vi "EtherNet_IP Scan Registers.vi"(4 "error in":errorcluster, 5 "No of Elements":u8, 6 "Offset(N7:?)":u8, 7 "Connection Cluster":T1={"TCP Connection"=refnum, "Session"=[], "EtherNet/IP Device Address"="172.20.37.243"} {"Session" format="0x%02x"}) -> (0 "error out":errorcluster, 1 "Data Error":bool, 2 "Registers":u16[](array[numeric]), 3 "Connection Cluster Out":T1)   [LabVIEW 2020, in "EtherNet_IP_Lib.lvlib"]
uses:
  EtherNet_IP_Lib.lvlib
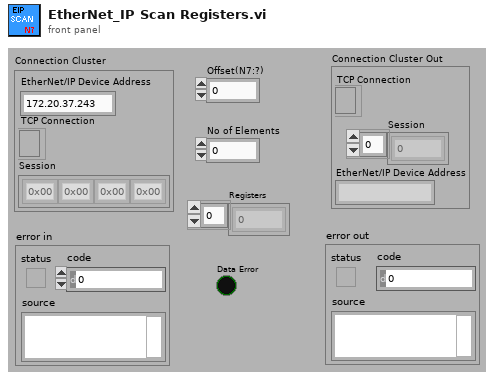
[diagram p1: front panel]
types:
  T1 = cluster{"TCP Connection":refnum<k5>, "Session":u8[], "EtherNet/IP Device Address":string}
  T2 = enum16{"Standard", "Buffered", "CRLF", "Immediate"}
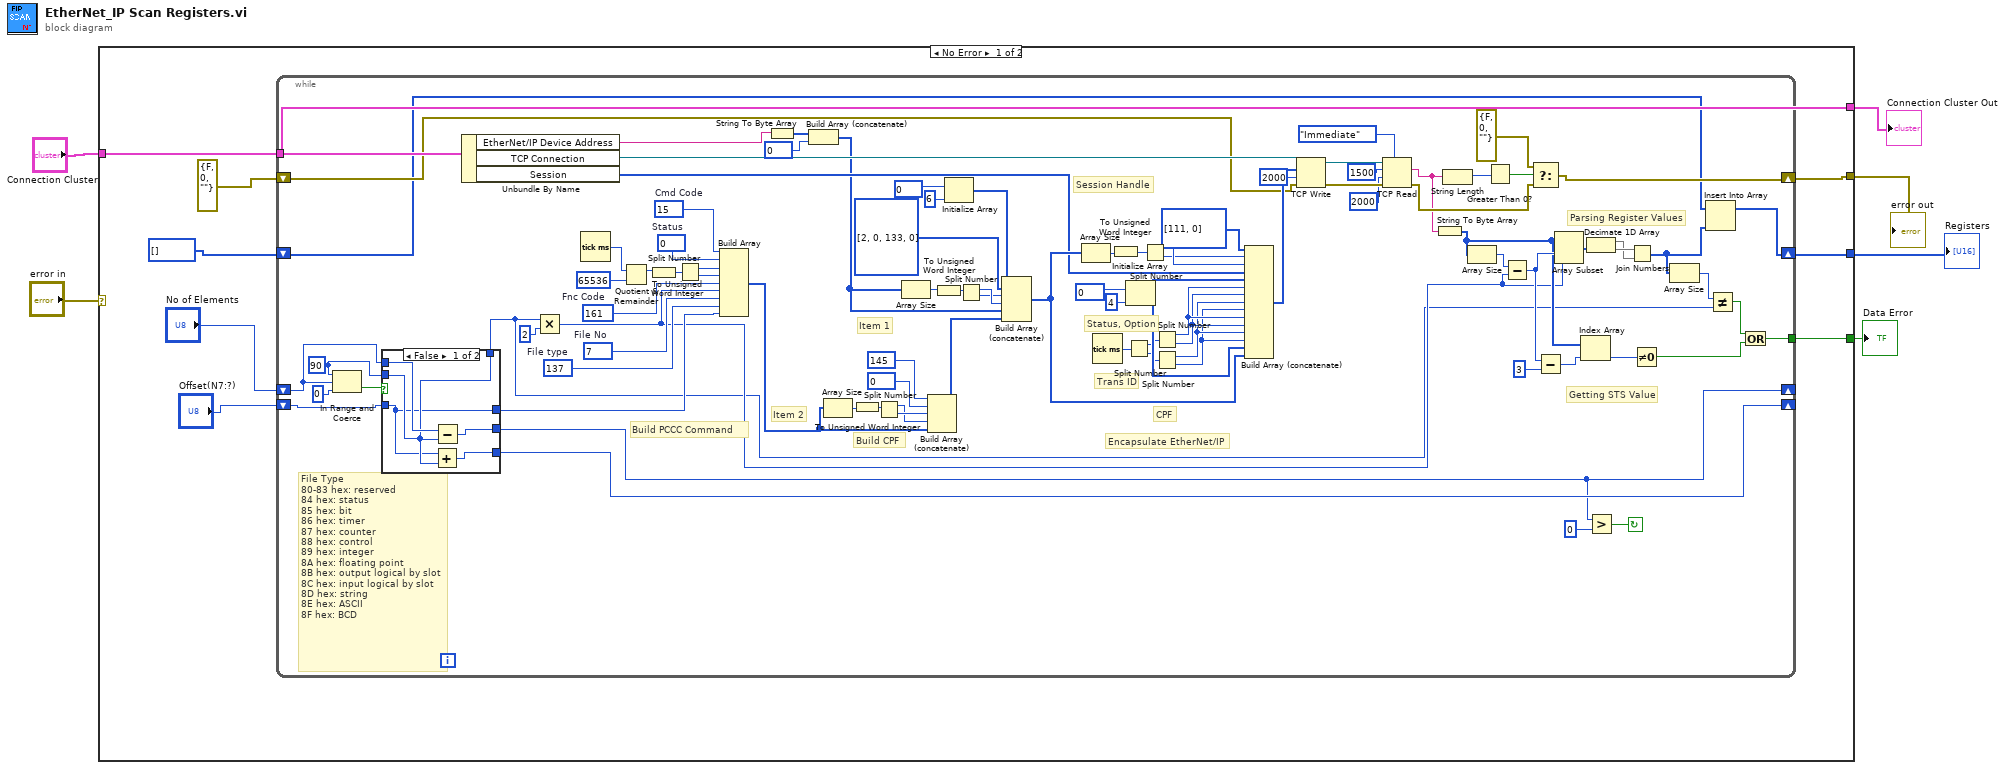
[diagram p0: block diagram]
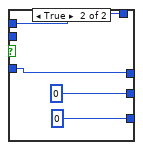
[diagram p2: hidden frame]
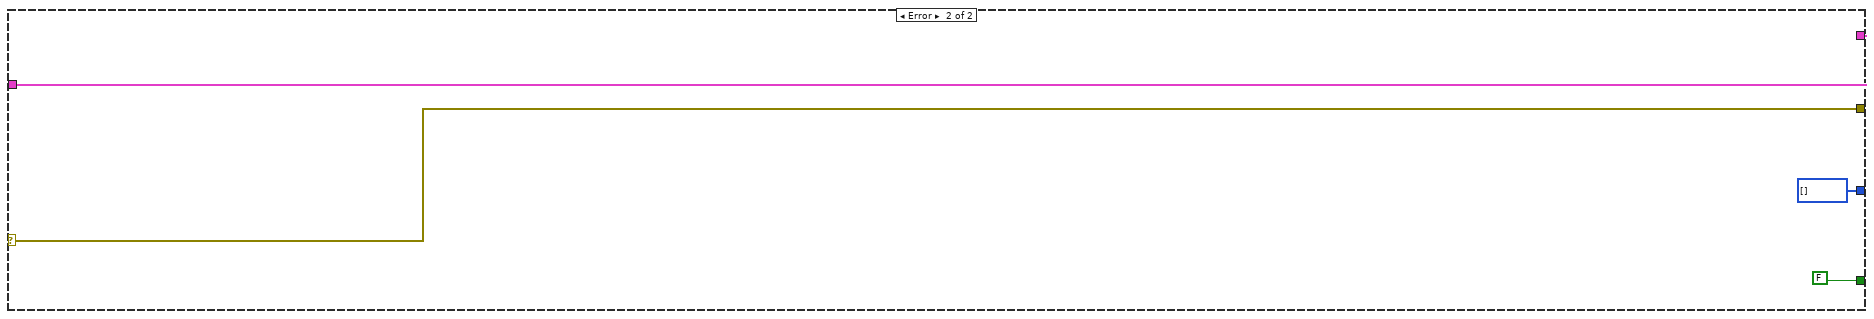
[diagram p3: hidden frame]
diagram:
  n1 = case shown="No Error" "error in" {
    selector: "error in" -> [_ w120]
    tunnel: "Connection Cluster" -> [w14 w119]
    tunnel: [w13 w120] -> w6
    tunnel: [w14 w119] -> w3
    tunnel: [w12 u16[] []] -> w2
    tunnel: [w11 FALSE] -> w1
    frame No Error {
      n2 = while {
        tunnel: w14 -> [w64]
        tunnel: [w32] -> w11
        shift-right: [w25] -> _
        shift-left: "No of Elements" -> [w28]
        shift-right: [w26] -> _
        shift-left: "Offset(N7:?)" -> [w27]
        shift-right: [w59] -> w13
        shift-left: errorcluster {"status"=FALSE, "code"=0, "source"=""} ("error out") -> [w21]
        shift-right: [w18] -> w12
        shift-left: u16[] [] -> [w19]
        stop <- w23 continue-if-true
        w22 = u8 90 ("upper limit")
        w50 = u8 137  # File type
        w51 = u8 7  # File No
        w52 = u8 161  # Fnc Code
        w100 = u8 0  # Status
        w99 = u8 15  # Cmd Code
        # "Getting STS Value"
        # "Parsing Register Values"
        # "File Type\n80-83 hex: reserved\n84 hex: status\n85 hex: bit\n86 hex: timer\n87 hex: counter\n88 hex: control\n89 hex: integer\n8A hex: floating point\n8B hex: output logical by slot\n8C hex: input logical by slot\n8D hex: string\n8E hex: ASCII\n8F hex: BCD"
        # "Build CPF"
        # "Trans ID"
        # "CPF"
        # "Status, Option"
        # "Session Handle"
        # "Item 2"
        # "Item 1"
        # "Encapsulate EtherNet/IP"
        # "Build PCCC Command"
        n3 = In Range and Coerce(upper limit=w22, x=w28, lower limit=u8 0) -> (In Range?=w29:bool)  [unwired: 1 out]
        n4 = case shown="False" w29 {
          tunnel: w28 -> [w112 w115]
          tunnel: w27 -> [w109 w116]
          tunnel: [w109 w116] -> w17
          tunnel: [w110 w115] -> w15
          tunnel: [w111 u8 0] -> w25
          tunnel: [w108 u8 0] -> w26
          tunnel: w22 -> [w110 _]
          frame False {
            n5 = Add(x=w109, y=w110) -> (x+y=w108:u8)
            n6 = Subtract(x=w112, y=w110) -> (x-y=w111:u8)
          }
          frame True {
          }
        }
        n7 = Unbundle By Name(w64) -> ("EtherNet/IP Device Address"=w65:string, "TCP Connection"=w104:refnum<k5>, "Session"=w75:u8[])
        n8 = Multiply(x=w15, y=u8 2) -> (x*y=w16:u8)
        n9 = Tick Count (ms)() -> (millisecond timer value=w95:u32)
        n10 = Quotient & Remainder(x=w95, y=u32 65536) -> (x-y*floor(x/y)=w97:u32)  [unwired: 1 out]
        n11 = To Unsigned Word Integer(number=w97) -> (unsigned 16bit integer=w98:u16)
        n12 = Split Number(x=w98) -> (hi(x)=w101:u8, lo(x)=w102:u8)
        n13 = Build Array(w99, w100, w101, w102, w52, w16, w51, w50, w17) -> (w54:u8[])
        n14 = String To Byte Array(string=w65) -> (unsigned byte array=w93:u8[])
        n15 = Build Array (concatenate)(w93, u8 0 ("Status")) -> (w57:u8[])
        n16 = Array Size(array=w54) -> (size(s)=w92:i32)
        n17 = To Unsigned Word Integer(number=w92) -> (unsigned 16bit integer=w91:u16)
        n18 = Split Number(x=w91) -> (hi(x)=w89:u8, lo(x)=w90:u8)
        n19 = Array Size(array=w57) -> (size(s)=w55:i32)
        n20 = Build Array (concatenate)(u8 145 ("Status"), u8 0 ("Status"), w90, w89, w54) -> (w53:u8[])
        n21 = To Unsigned Word Integer(number=w55) -> (unsigned 16bit integer=w56:u16)
        n22 = Initialize Array(u8 0 ("Status"), 6 ("dimension size")) -> (w84:u8[])
        n23 = Split Number(x=w56) -> (hi(x)=w47:u8, lo(x)=w46:u8)
        n24 = Build Array (concatenate)(w84, u8[] [2, 0, 133, 0], w46, w47, w57, w53) -> (w76:u8[])
        n25 = Array Size(array=w76) -> (size(s)=w82:i32)
        n26 = Tick Count (ms)() -> (millisecond timer value=w74:u32)
        n27 = To Unsigned Word Integer(number=w82) -> (unsigned 16bit integer=w83:u16)
        n28 = Split Number(x=w74) -> (hi(x)=w73:u16, lo(x)=w72:u16)
        n29 = Initialize Array(u8 0 ("Status"), 4 ("dimension size")) -> (w77:u8[])
        n30 = Split Number(x=w83) -> (hi(x)=w81:u8, lo(x)=w80:u8)
        n31 = Split Number(x=w73) -> (hi(x)=w71:u8, lo(x)=w70:u8)
        n32 = Split Number(x=w72) -> (hi(x)=w69:u8, lo(x)=w68:u8)
        n33 = Build Array (concatenate)(u8[] [111, 0], w80, w81, w75, w77, w71, w70, w69, w68, w71, w70, w69, w68, w77, w76) -> (w67:u8[])
        n34 = TCP Write(connection ID=w104, data in=w67, error in (no error)=w21, 9:2000 ("timeout ms (25000)")) -> (connection ID out=w106:refnum<k5>, error out=w107:errorcluster)  [unwired: 1 out]
        n35 = TCP Read(connection ID=w106, bytes to read=1500, error in (no error)=w107, 7:T2."Immediate" ("mode (standard)"), 9:2000 ("timeout ms (25000)")) -> (data out=w58:string, error out=w60:errorcluster)  [unwired: 1 out]
        n36 = String To Byte Array(string=w58) -> (unsigned byte array=w36:u8[])
        n37 = String Length(string=w58) -> (length=w63:i32)
        n38 = Array Size(array=w36) -> (size(s)=w44:i32)
        n39 = Greater Than 0?(x=w63) -> (x > 0?=w62:bool)
        n40 = Subtract(x=w44, y=w16) -> (x-y=w39:i32)
        n41 = Select(t=errorcluster {"status"=FALSE, "code"=0, "source"=""} ("error IO"), s=w62, f=w60) -> (s? t:f=w59:errorcluster)
        n42 = Subtract(x=w39, y=3) -> (x-y=w37:i32)
        n43 = Array Subset(array=w36, index=w39, length=w16) -> (w43:u8[])
        n44 = Index Array(array=w36, index=w37) -> (element=w35:u8)
        n45 = Decimate 1D Array(w43) -> (w41:u8[], w42:u8[])
        n46 = Greater?(x=w25, y=u8 0) -> (0:w23:bool)
        n47 = Join Numbers(hi=w42, lo=w41) -> ((hi.lo)=w20:u16[])
        n48 = Not Equal To 0?(x=w35) -> (x != 0?=w33:bool)
        n49 = Array Size(array=w20) -> (size(s)=w40:i32)
        n50 = Insert Into Array(array=w19, new element=w20) -> (w18:u16[])  [unwired: 1 in]
        n51 = Not Equal?(x=w40, y=w15) -> (x != y?=w34:bool)
        n52 = Or(x=w34, y=w33) -> (x .or. y?=w32:bool)
      }
    }
    frame Error {
    }
  }
  "error out" <- w6
  "Connection Cluster Out" <- w3
  "Registers" <- w2
  "Data Error" <- w1
